vi "heatmap.vi"(1 "Ranges":i32[](array[numeric]), 2 "Colorset":u32[](array[numeric]), 3 "Temp 1D":dbl[](array[numeric])) -> (0 "2D Heatmap":u32[][](array[numeric]))   [LabVIEW 2017]
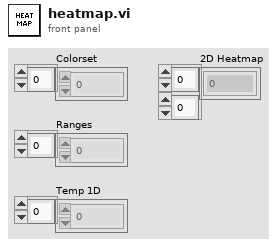
[diagram p1: front panel]
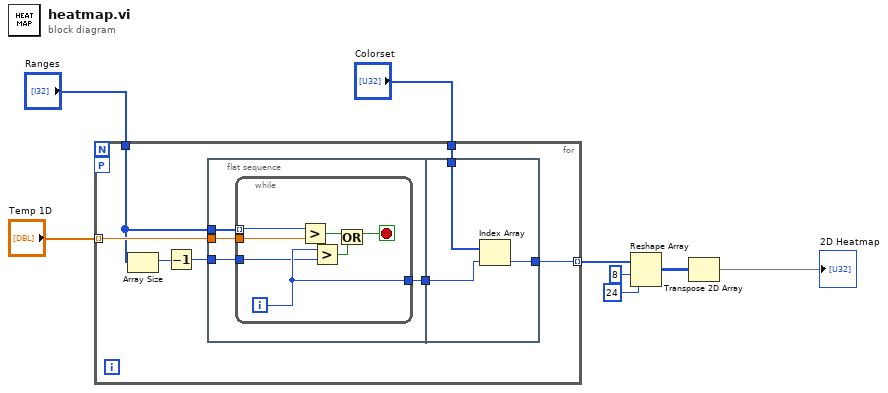
[diagram p0: block diagram]
diagram:
  n1 = for {
    tunnel: "Temp 1D" -> [w15] mode=indexing
    workers-P: _ -> [_]
    tunnel: "Colorset" -> [w14]
    tunnel: "Ranges" -> [w11]
    tunnel: [w12] -> w7 mode=indexing
    n2 = Array Size(array=w11) -> (size(s)=w10:i32)
    n3 = Decrement(x=w10) -> (x-1=w9:i32)
    n4 = flat-sequence {
      tunnel: w15 -> [w19]
      tunnel: w11 -> [w18]
      tunnel: [w17] -> w13
      tunnel: w9 -> [w16]
      tunnel: w14 -> [w29]
      tunnel: w13 -> [w28]
      tunnel: [w27] -> w12
      frame #0 {
        n5 = while {
          tunnel: w19 -> [w26]
          tunnel: w18 -> [w25] mode=indexing
          tunnel: [w21] -> w17
          tunnel: w16 -> [w20]
          i -> [w21]
          stop <- w24 stop-if-true
          n6 = Greater?(x=w25, y=w26) -> (0:w23:bool)
          n7 = Greater?(x=w21, y=w20) -> (0:w22:bool)
          n8 = Or(x=w23, y=w22) -> (x .or. y?=w24:bool)
        }
      }
      frame #1 {
        n9 = Index Array(array=w29, index=w28) -> (element=w27:u32)
      }
    }
  }
  n10 = Reshape Array(w7, 8 ("dimension size"), 24 ("dimension size")) -> (w4:u32[][])
  n11 = Transpose 2D Array(2D array=w4) -> (transposed array=→"2D Heatmap":u32[][])
